vi "Error Display Window (Main).vi"(8 "Error In":errorcluster, 11 "New Error Details":T1) -> (0 "Error Out":errorcluster)   [LabVIEW 2023, in "Error Manager.lvlib" / "Error Display Window.lvclass"]
doc: "This is a user-facing window that displays to the user the error code, error message, and timestamp of a LabVIEW error that occured in the application.\n\n<B>Note</B>: Not necessarily every error that occurs in an application will be displayed by this dialogue. For example, if a while loop in an application starts producing the same error in a loop, and starts \"spamming\" the Error Manager module with dozens or hundreds of errors every second, if would be undesirable to popup this window once for every such error."
uses:
  Error Display Window.lvclass
  Error Details (cluster).ctl
  Private VIs/Close Window Option (Enum).ctl
  <vilib>/Utility/error.llb/DialogType.ctl
  Error Display Window.lvclass/Error Display Window.ctl
  Error Manager.lvlib
  Settings/Settings.lvclass
panel:
  out "Error Message":string
  out "Error Code":i32
  in  "Sizing Tool":bool
  in  "OK Button":bool
  out "EHL iteration":i32
  out "Pre-loop Init":errorcluster
  # "User-facing region."
  # "Error"
  # "Non-user-facing region. Developer-facing only."
  # "Input\nInputs to the VI"
  # "Development\ncontrols/indicators useful for development and testing, but which are not outputs of the VI"
  # "Output\nOutputs of the VI"
  # "The Error Out indicator is larger than usual in order to be able to view the full error message without having to scroll."
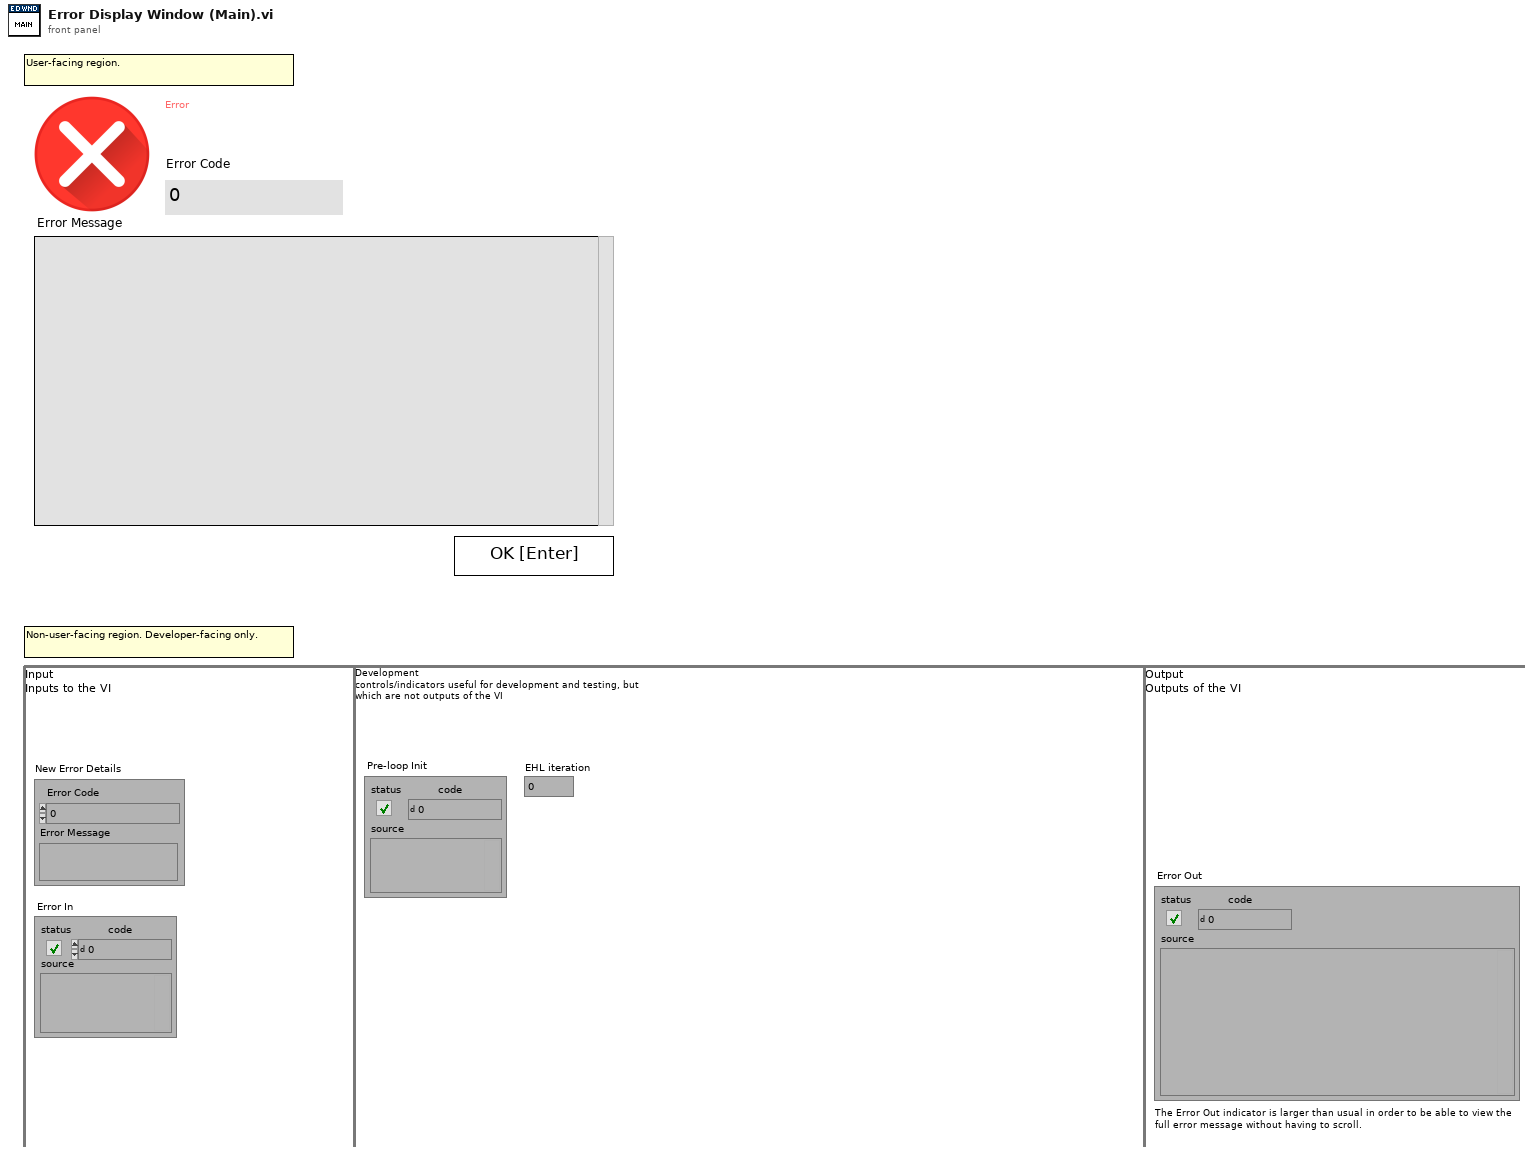
[diagram p1: front panel]
types:
  T1 = typedef "Error Manager.lvlib/Error Display Window.lvclass/Error Details (cluster).ctl" = cluster{"Error Code":i32, "Error Message":string}
  T2 = typedef "Error Manager.lvlib/Close Window Option (Enum).ctl" = enum16{"In dev env, don't close", "In dev env, don't close if top-level caller", "Close Always"}
  T3 = typedef "Error Manager.lvlib/Settings.lvclass/Window_Behaviour (enum).ctl" = enum16{"Default", "Floating", "Modal"}
  T4 = typedef "DialogType.ctl" = u16
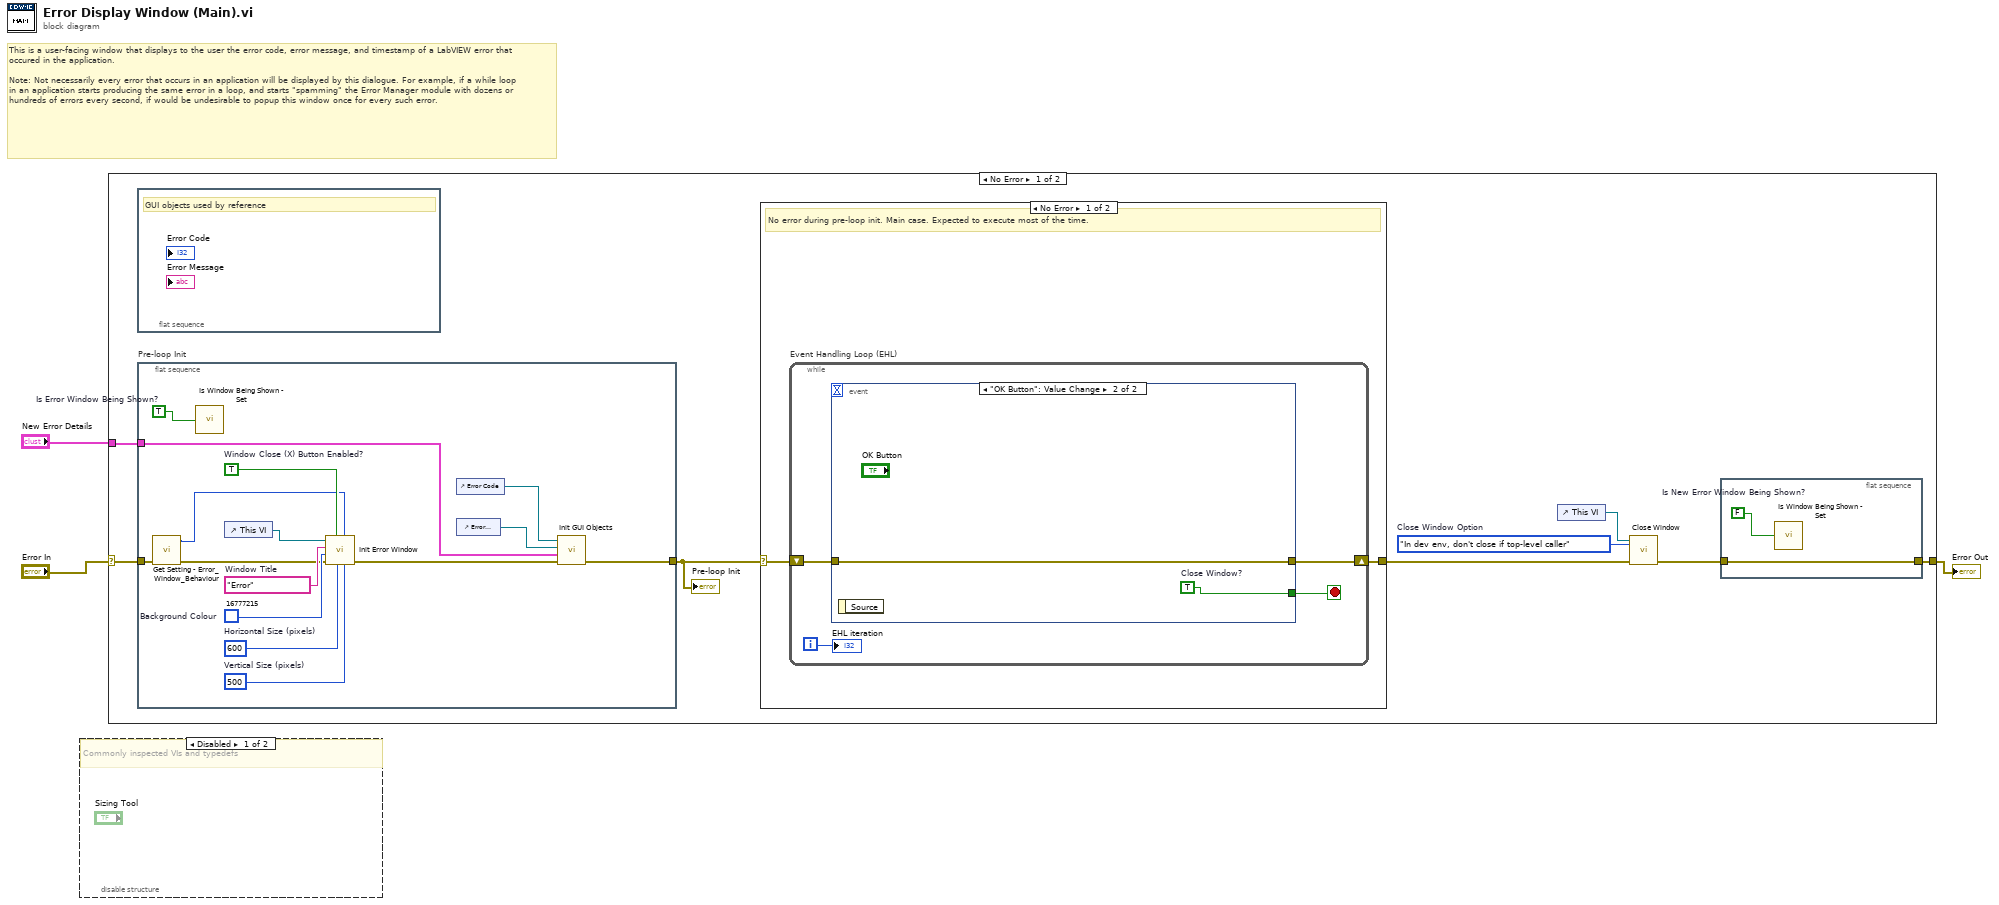
[diagram p0: block diagram]
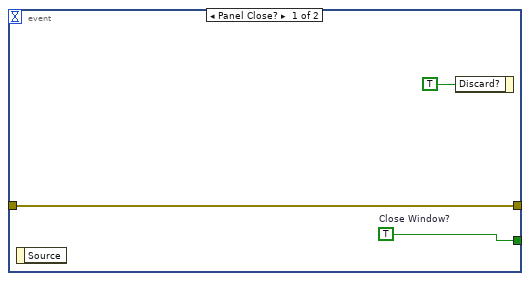
[diagram p2: hidden frame]
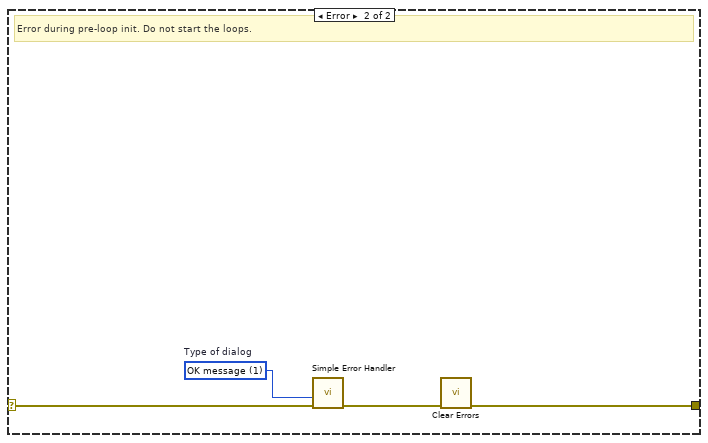
[diagram p3: hidden frame]
diagram:
  # "This is a user-facing window that displays to the user the error code, error message, and timestamp of a LabVIEW error that occured in the application.\n\nNote: Not necessarily every error that occurs in an application will be displayed by this dialogue. For example, if a while loop in an application starts producing the same error in a loop, and starts \"spamming\" the Error Manager module with dozens or hundreds of errors every second, if would be undesirable to popup this window once for every such error."
  n1 = disable-structure shown="Disabled" {
    frame Disabled {
      # "Commonly inspected VIs and typedefs"
    }
    frame Enabled {
    }
  }
  n2 = case shown="No Error" "Error In" {
    selector: "Error In" -> [w10 w44]
    tunnel: [w9 w44] -> w3
    tunnel: "New Error Details" -> [w8 _]
    frame No Error {
      w4 = Close_Window_Option_(Enum)."In dev env, don't close if top-level caller"  # Close Window Option
      n3 = flat-sequence {
        frame #0 {
          # "GUI objects used by reference"
        }
      }
      n4 = flat-sequence "Pre-loop Init" {
        tunnel: [w20] -> w11
        tunnel: w10 -> [w21]
        tunnel: w8 -> [w18]
        frame #0 {
          w16 = TRUE  # Window Close (X) Button Enabled?
          w17 = u32 16777215  # Background Colour
          w24 = i16 500  # Vertical Size (pixels)
          w23 = i16 600  # Horizontal Size (pixels)
          w22 = "Error"  # Window Title
          w28 = TRUE  # Is Error Window Being Shown?
          n5 = call "Get Setting - Error_Window_Behaviour.vi"("Error In"=w21) -> ("Error Out"=w15:errorcluster, "Error_Window_Behaviour"=w14:T3)  [unwired: 9 in]
          n6 = call "Is Window Being Shown - Set.vi"("Is Window Being Shown?"=w28) -> ()
          n7 = control-ref of="This VI"() -> (w25:refnum<vi>)
          n8 = call "Init Error Window.vi"("Window Vertical Size (pixels)"=w24, "Window Behaviour"=w14, "Window Horizontal Size (pixels)"=w23, "Window Close (X) Button Enabled? (Default = True)"=w16, "error in"=w15, "Background Colour (Default = 255,255,255)"=w17, "Window Title"=w22, "VI Refnum"=w25) -> ("error out"=w19:errorcluster)  [unwired: 3 in]
          n9 = control-ref of="Error Code"() -> (w27:refnum<vi>)
          n10 = control-ref of="Error Message"() -> (w26:refnum<vi>)
          n11 = call "Init GUI Objects.vi"("error in"=w19, "New Error"=w18, "Error Message"=w26, "Error Code"=w27) -> ("error out"=w20:errorcluster)  [unwired: 7 in]
        }
      }
      n12 = case shown="No Error" w11 {
        selector: w11 -> [w29 w43]
        tunnel: [w30 w41] -> w6
        frame No Error {
          # "No error during pre-loop init. Main case. Expected to execute most of the time."
          n13 = while "Event Handling Loop (EHL)" {
            shift-right: [w32] -> w30
            shift-left: w29 -> [w34]
            i -> [w31]
            stop <- w33 stop-if-true
            n14 = event shown="[1] \"OK Button\": Value Change" {
              selector: _ -> [_ _]
              dyn-events: _ -> [_ _]
              timeout: _ -> [_ _]
              tunnel: w34 -> [w36 w39]
              tunnel: [w35 w38] -> w33
              tunnel: [w36 w39] -> w32
              event Panel Close? {
                w35 = TRUE  # Close Window?
                n15 = event-data() -> ()  [unwired: 1 in, 1 out]
                n16 = event-data("Discard?"=TRUE) -> ()  [unwired: 1 in, 1 out]
              }
              event "OK Button": Value Change {
                w38 = TRUE  # Close Window?
                n17 = event-data() -> ()  [unwired: 1 in, 1 out]
              }
            }
            "EHL iteration" <- w31
          }
        }
        frame Error {
          w40 = T4 1 items=["no dialog", "OK message", "continue or stop message", "OK message + warnings", "continue/stop + warnings"]  # Type of dialog
          # "Error during pre-loop init. Do not start the loops."
          n18 = call <vilib>:"Simple Error Handler.vi"("type of dialog (OK msg:1)"=w40, "error in (no error)"=w43) -> ("error out"=w42:errorcluster)  [unwired: 3 in, 4 out]
          n19 = call <vilib>:"Clear Errors.vi"("error in (no error)"=w42) -> ("error out"=w41:errorcluster)  [unwired: 5 in, 1 out]
        }
      }
      n20 = control-ref of="This VI"() -> (w7:refnum<vi>)
      n21 = call "Close Window.vi"("error in"=w6, "Close Window Option (Default = \"In dev env, don't close if top-level caller\")"=w4, "VI Refnum"=w7) -> ("error out"=w5:errorcluster)  [unwired: 8 in]
      n22 = flat-sequence {
        tunnel: [w13] -> w9
        tunnel: w5 -> [w13]
        frame #0 {
          w12 = FALSE  # Is New Error Window Being Shown?
          n23 = call "Is Window Being Shown - Set.vi"("Is Window Being Shown?"=w12) -> ()
        }
      }
      "Pre-loop Init" <- w11
    }
    frame Error {
      # "Error upstream. Do nothing."
    }
  }
  "Error Out" <- w3
